vi "wheel.vi"(8 "에러 입력":errorcluster, 9 "R_pwm":i32, 10 "L_pwm":i32, 11 "FPGA VI 참조 입력":refnum<k20>) -> (0 "에러 출력":errorcluster, 3 "FPGA VI 참조 출력":refnum<k20>)   [LabVIEW 2019]
uses:
  <vilib>/Platform/TimedLoop/XDataNode/timing_clust.ctl
  <vilib>/Platform/TimedLoop/XDataNode/nitl_modes.ctl
  <vilib>/Platform/TimedLoop/XDataNode/wakeup.ctl
  <vilib>/Utility/error.llb/Error Cluster From Error Code.vi
  <vilib>/rvi/errors/niLvFpgaAdjustHostInterfaceError.vi
  global_stop.vi
  <vilib>/rvi/interface/nirviReadWriteControl/nirviReadWriteControl.xnode
  <vilib>/Platform/TimedLoop/XDataNode/XDataNode.xnode
  <vilib>/Platform/TimedLoop/XDataNode/XDNodeRunTimeDep.lvlib
  <vilib>/rvi/interface/Simulation/niFpgaSimulationCallBeginRW.vi
  NiFpgaLv.dll
panel:
  out "mm/ms":dbl
  in  "R_dir":bool
  in  "L_dir":bool
  out "R_이동 거리":dbl
  out "R_Encoder":i32
  in  "wheel_stop":bool
  out "타임아웃":i32
  out "L_이동 거리":dbl
  out "L_encoder":i32
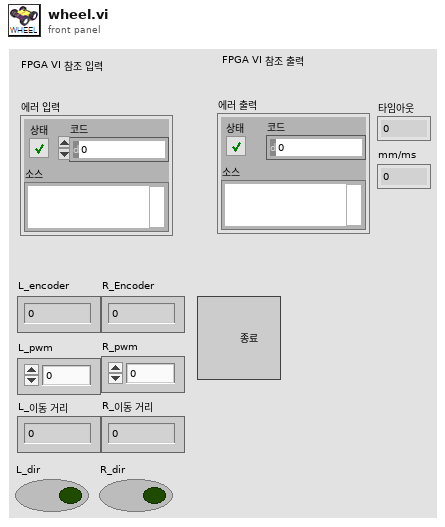
[diagram p1: front panel]
types:
  T1 = typedef "XDNodeRunTimeDep.lvlib/timing_clust.ctl" = cluster{"Expected End [f-1]":u64, "Actual End [f-1]":u64, "Finished Late? [f-1]":bool, "Expected End [i-1]":u64, "Actual End [i-1]":u64, "Finished Late? [i-1]":bool, "Expected Start [i]":u64, "Actual Start [i]":u64, "Expected Start [f]":u64, "Actual Start [f]":u64, "Source Name":string, "Structure Name":string, "Period":i64, "Deadline":i64, "Offset":i64, "Start":i64, "Priority":i32, "Timeout":i32, "Mode":T2, "Wakeup Reason":T3, "Error":errorcluster, "Source Type":string, "Secondary Source Type":string, "Global End Time":u64, "Global Start Time":u64, "Frame Duration":u64, "Iteration Duration":u64, "Assigned CPU":i32, "I/O Scan Engine Mode":u32}
  T2 = typedef "XDNodeRunTimeDep.lvlib/nitl_modes.ctl" = enum32{"No Change", "Process missed periods, maintain original phase", "Discard missed periods, maintain original phase", "Process missed periods, ignore original phase", "Discard missed periods, ignore original phase"}
  T3 = typedef "XDNodeRunTimeDep.lvlib/wakeup.ctl" = enum32{"Normal", "Aborted", "Asynchronous wakeup", "Timing source error", "Timed loop error", "Timeout"}
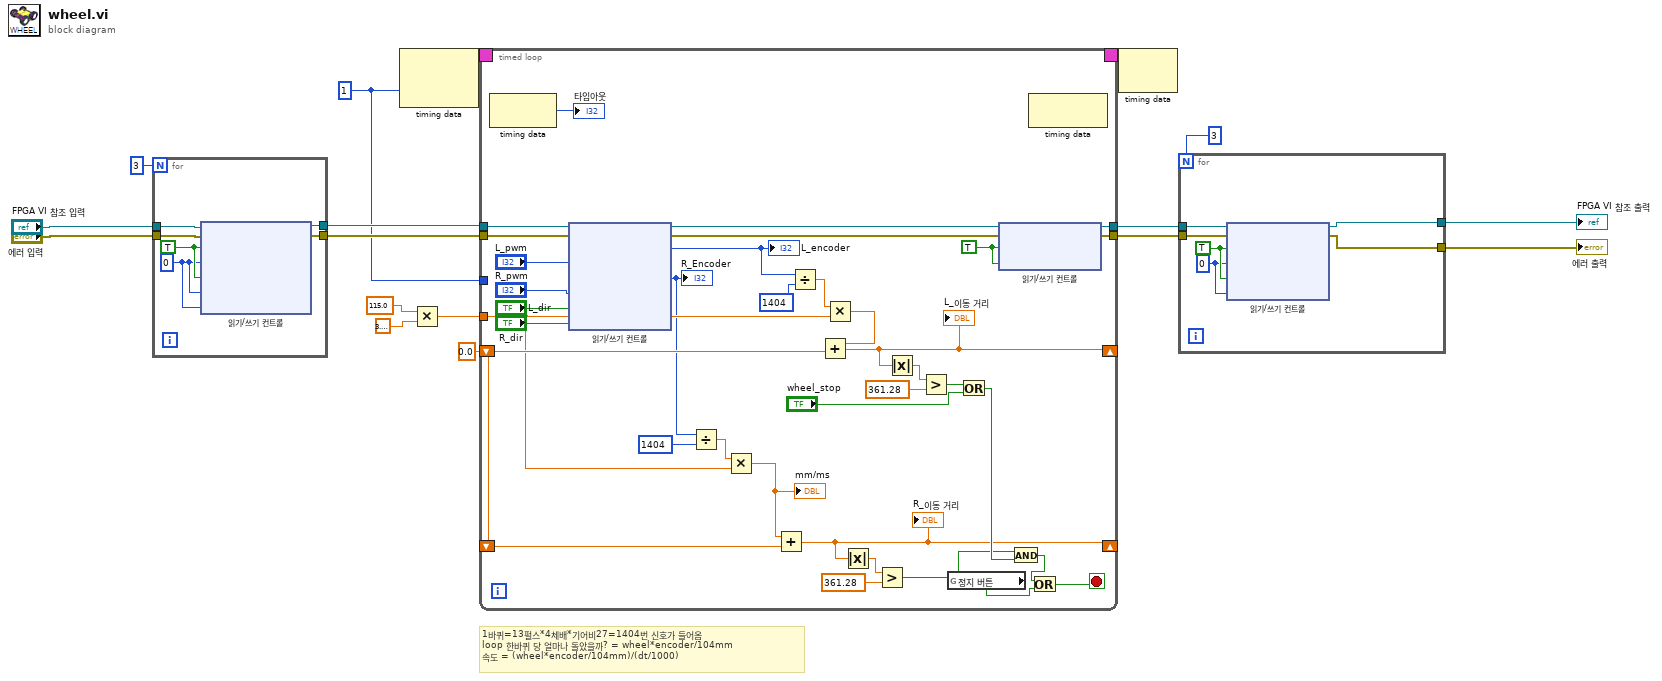
[diagram p0: block diagram]
diagram:
  w5 = 0.0
  w6 = i64 1 ("주기")
  # "1바퀴=13펄스*4체배*기어비27=1404번 신호가 들어옴\nloop 한바퀴 당 얼마나 돌았을까? = wheel*encoder/104mm\n속도 = (wheel*encoder/104mm)/(dt/1000)"
  n1 = for {
    N: 3 -> [_]
    tunnel: [w23] -> w14
    tunnel: [w22] -> w13
    tunnel: "에러 입력" -> [w19]
    tunnel: "FPGA VI 참조 입력" -> [w18]
    w20 = 0 ("pwm input(escon)")
    w21 = TRUE ("encoder reset")
    n2 = xnode "읽기/쓰기 컨트롤"("FPGA VI 참조 입력"=w18, "에러 입력"=w19, "encoder reset"=w21, "pwm input"=w20, "R_encoder reset"=w21, "R_pwm input"=w20, "직동_pwm input"=w20) -> ("FPGA VI 참조 출력"=w23:refnum<k20>, "에러 출력"=w22:errorcluster)
  }
  n3 = node-c288(w6) -> (w17:T1)  [unwired: 1 in]
  n4 = Multiply(x=115.0, y=3.141592653589793) -> (x*y=w7:dbl)
  n5 = timed-loop {
    timing: w17 -> [_]
    timing-out: [_] -> w16
    tunnel: w14 -> [w41]
    tunnel: w13 -> [w40]
    tunnel: [w54] -> w12
    tunnel: [w53] -> w11
    tunnel: w7 -> [w39]
    tunnel: w6 -> [_]
    shift-right: [w44] -> _
    shift-left: w5 -> [w50]
    shift-right: [w38] -> _
    shift-left: w5 -> [w37]
    stop <- w26 stop-if-true
    w43 = TRUE ("encoder reset")
    n6 = node-c288() -> (→"타임아웃":i32)  [unwired: 1 in]
    n7 = xnode "읽기/쓰기 컨트롤"("FPGA VI 참조 입력"=w41, "에러 입력"=w40, "pwm input"="L_pwm", "R_pwm input"="R_pwm", "L_dir"="L_dir", "R_dir"="R_dir") -> ("FPGA VI 참조 출력"=w56:refnum<k20>, "에러 출력"=w55:errorcluster, "Encoder  (4x)"=w58:i32, "R_Encoder  (4x)"=w35:i32)
    "L_encoder" <- w58
    "R_Encoder" <- w35
    n8 = Divide(x=w35, y=1404) -> (x/y=w31:dbl)
    n9 = Multiply(x=w31, y=w39) -> (x*y=w33:dbl)
    "mm/ms" <- w33
    n10 = Add(x=w33, y=w37) -> (x+y=w38:dbl)
    "R_이동 거리" <- w38
    n11 = Divide(x=w58, y=1404) -> (x/y=w48:dbl)
    n12 = Multiply(x=w48, y=w39) -> (x*y=w51:dbl)
    n13 = Add(x=w51, y=w50) -> (x+y=w44:dbl)
    "L_이동 거리" <- w44
    n14 = Absolute Value(x=w38) -> (abs(x)=w29:dbl)
    n15 = Greater?(x=w29, y=361.28) -> (0:w30:bool)
    n16 = Absolute Value(x=w44) -> (abs(x)=w45:dbl)
    n17 = Greater?(x=w45, y=361.28) -> (0:w47:bool)
    n18 = global read "global_stop.vi" "정지 버튼"() -> (w24:bool)
    n19 = Or(x=w47, y="wheel_stop") -> (x .or. y?=w42:bool)
    n20 = xnode "읽기/쓰기 컨트롤"("FPGA VI 참조 입력"=w56, "에러 입력"=w55, "encoder reset"=w43, "R_encoder reset"=w43) -> ("FPGA VI 참조 출력"=w54:refnum<k20>, "에러 출력"=w53:errorcluster)
    n21 = And(x=w30, y=w42) -> (x .and. y?=w25:bool)
    n22 = node-c288() -> ()  [unwired: 1 in, 1 out]
    n23 = Or(x=w25, y=w24) -> (x .or. y?=w26:bool)
  }
  n24 = node-c288(w16) -> ()  [unwired: 1 out]
  n25 = for {
    N: 3 -> [_]
    tunnel: w12 -> [w68]
    tunnel: w11 -> [w67]
    tunnel: [w64] -> w4
    tunnel: [w63] -> w3
    w65 = 0 ("pwm input(escon)")
    w66 = TRUE ("encoder reset")
    n26 = xnode "읽기/쓰기 컨트롤"("FPGA VI 참조 입력"=w68, "에러 입력"=w67, "encoder reset"=w66, "pwm input"=w65, "R_encoder reset"=w66, "R_pwm input"=w65) -> ("FPGA VI 참조 출력"=w63:refnum<k20>, "에러 출력"=w64:errorcluster)
  }
  "FPGA VI 참조 출력" <- w3
  "에러 출력" <- w4
